vi "WriteLine.vi"(8 "Error In":errorcluster, 10 "ConsoleText":string) -> (0 "Error Out":errorcluster)   [LabVIEW 2020, in "Console.lvclass"]
uses:
  Console.lvclass
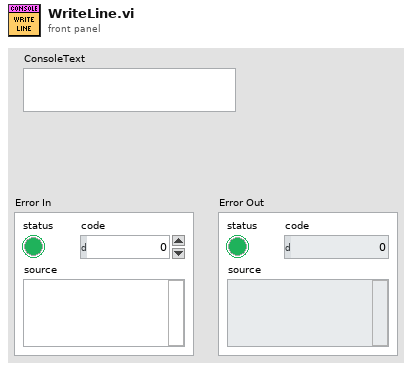
[diagram p1: front panel]
types:
  T1 = typedef "Console.lvclass/ObjectAttributes.ctl" = cluster{"ConsoleText":string[]}
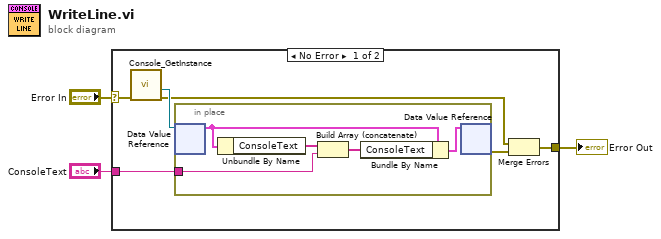
[diagram p0: block diagram]
diagram:
  n1 = case shown="No Error" "Error In" {
    selector: "Error In" -> [w8 w15]
    tunnel: [w9 w15] -> w2
    tunnel: "ConsoleText" -> [w4 _]
    frame No Error {
      n2 = call "Console_GetInstance.vi"("error in"=w8) -> ("error out"=w6:errorcluster, "DVRRefOut"=w7:refnum<data-value>)  [unwired: 6 in, 3 out]
      n3 = in-place {
        in-place-border: w4 -> [w10]
        n4 = in-place-dvr #1(w7) -> (w13:T1)  [unwired: 1 out]
        n5 = Unbundle By Name(w13) -> ("ConsoleText"=w12:string[])
        n6 = Build Array (concatenate)(w12, w10) -> (w11:string[])
        n7 = Bundle By Name(cluster=w13, "ConsoleText"=w11) -> (w14:T1)
        n8 = in-place-dvr #1(w14) -> (w5:errorcluster)  [unwired: 1 out]
      }
      n9 = Merge Errors(w6, w5) -> (w9:errorcluster)
    }
    frame Error {
    }
  }
  "Error Out" <- w2
